vi "F Dwf Digital In Buffer Size Info.vi"(8 "error in (no error)":errorcluster, 10 "pnSizeMax":i32, 11 "hdwf":i32) -> (0 "error out":errorcluster, 2 "pnSizeMax out":i32, 3 "function return":i32)   [LabVIEW 2021, in "Olasdwf.lvlib"]
doc: "DWFAPI int FDwfDigitalInBufferSizeInfo(HDWF hdwf, int *pnSizeMax);"
uses:
  Olasdwf.lvlib
  Windows/System32/dwf.dll
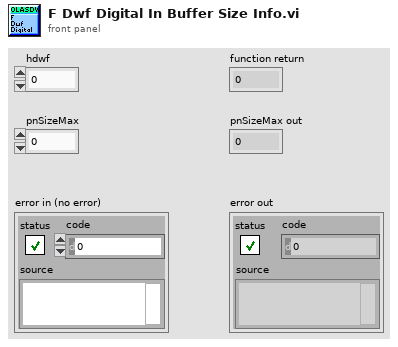
[diagram p1: front panel]
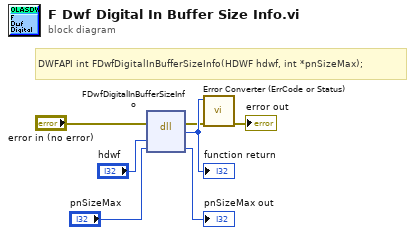
[diagram p0: block diagram]
diagram:
  # "DWFAPI int FDwfDigitalInBufferSizeInfo(HDWF hdwf, int *pnSizeMax);"
  n1 = dll-call lib="/Windows/System32/dwf.*" fn="FDwfDigitalInBufferSizeInfo"(error in="error in (no error)", "hdwf"="hdwf", "pnSizeMax"="pnSizeMax") -> (error out=w2:errorcluster, w7:i32, "pnSizeMax"=→"pnSizeMax out":i32)  [unwired: 3 in, 1 out]
  "function return" <- w7
  n2 = call "Error Converter (ErrCode or Status).vi"("error in (no error)"=w2, "error code"=w7) -> ("error out"=→"error out":errorcluster)  [unwired: 9 in]
